vi "Write 32-bit first word low.vi"(8 "error in (no error)":errorcluster, 10 "32-bit: first word low":bool, 11 "Modbus Module configuration in":refnum<class "Modbus Module configuration.lvclass">) -> (0 "error out":errorcluster, 3 "Modbus Module configuration.lvclass:Write 32-bit_ first word low.viModbus Module configuration out":refnum<class "Modbus Module configuration.lvclass">)   [LabVIEW 2015, in "Modbus Module configuration.lvclass"]
uses:
  Modbus Module configuration.lvclass
  Modbus Module configuration.lvclass/Modbus Module configuration.ctl
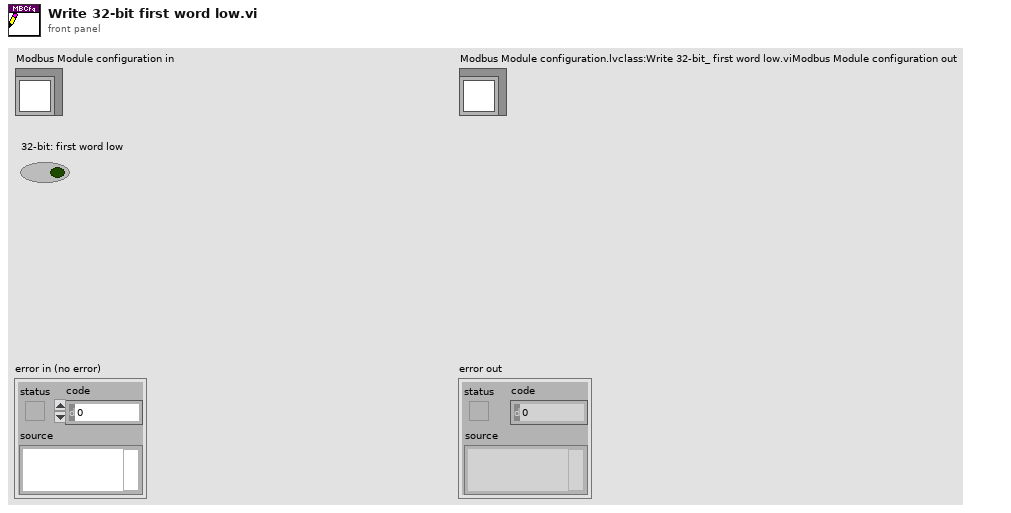
[diagram p1: front panel]
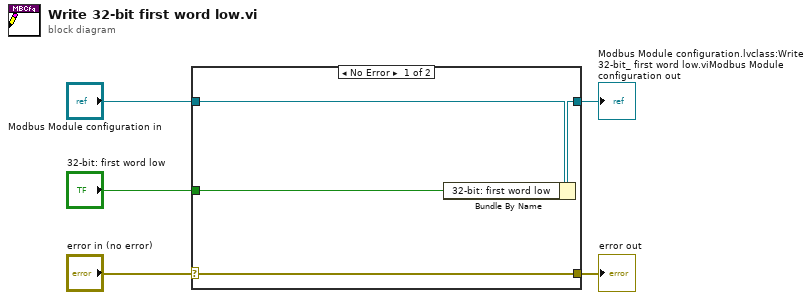
[diagram p0: block diagram]
diagram:
  n1 = case shown="No Error" "error in (no error)" {
    selector: "error in (no error)" -> [w9 w10]
    tunnel: [w9 w10] -> w4
    tunnel: [w7 w11] -> w2
    tunnel: "Modbus Module configuration in" -> [w8 w11]
    tunnel: "32-bit: first word low" -> [w6 _]
    frame No Error {
      n2 = Bundle By Name(cluster=w8, "32-bit: first word low"=w6) -> (w7:refnum<class "Modbus Module configuration.lvclass">)
    }
    frame Error {
    }
  }
  "error out" <- w4
  "Modbus Module configuration.lvclass:Write 32-bit_ first word low.viModbus Module configuration out" <- w2
